vi "Lissajous profiles.vi"() -> ()   [LabVIEW 2021]
panel:
  out "Sine":dynamicdata(graph)
  out "Variance":dynamicdata(graph)
  out "Standard Dev":dynamicdata(graph)
  out "Arithmetic Mean":dynamicdata(graph)
  in  "stop":bool
  in  "Amplitude 2":i32(knob) scale=0.0..10.0
  in  "Amplitude":i32(knob) scale=0.0..10.0
  in  "Phase 2":i32(knob) scale=0.0..50.0
  in  "Phase":i32(knob) scale=0.0..50.0
  in  "Frequency 2":i32(knob) scale=0.0..50.0
  in  "Frequency":i32(knob) scale=0.0..50.0
  out "Lissajous Graph":cluster{"Y":dbl[], "Y":dbl[]}[](graph)
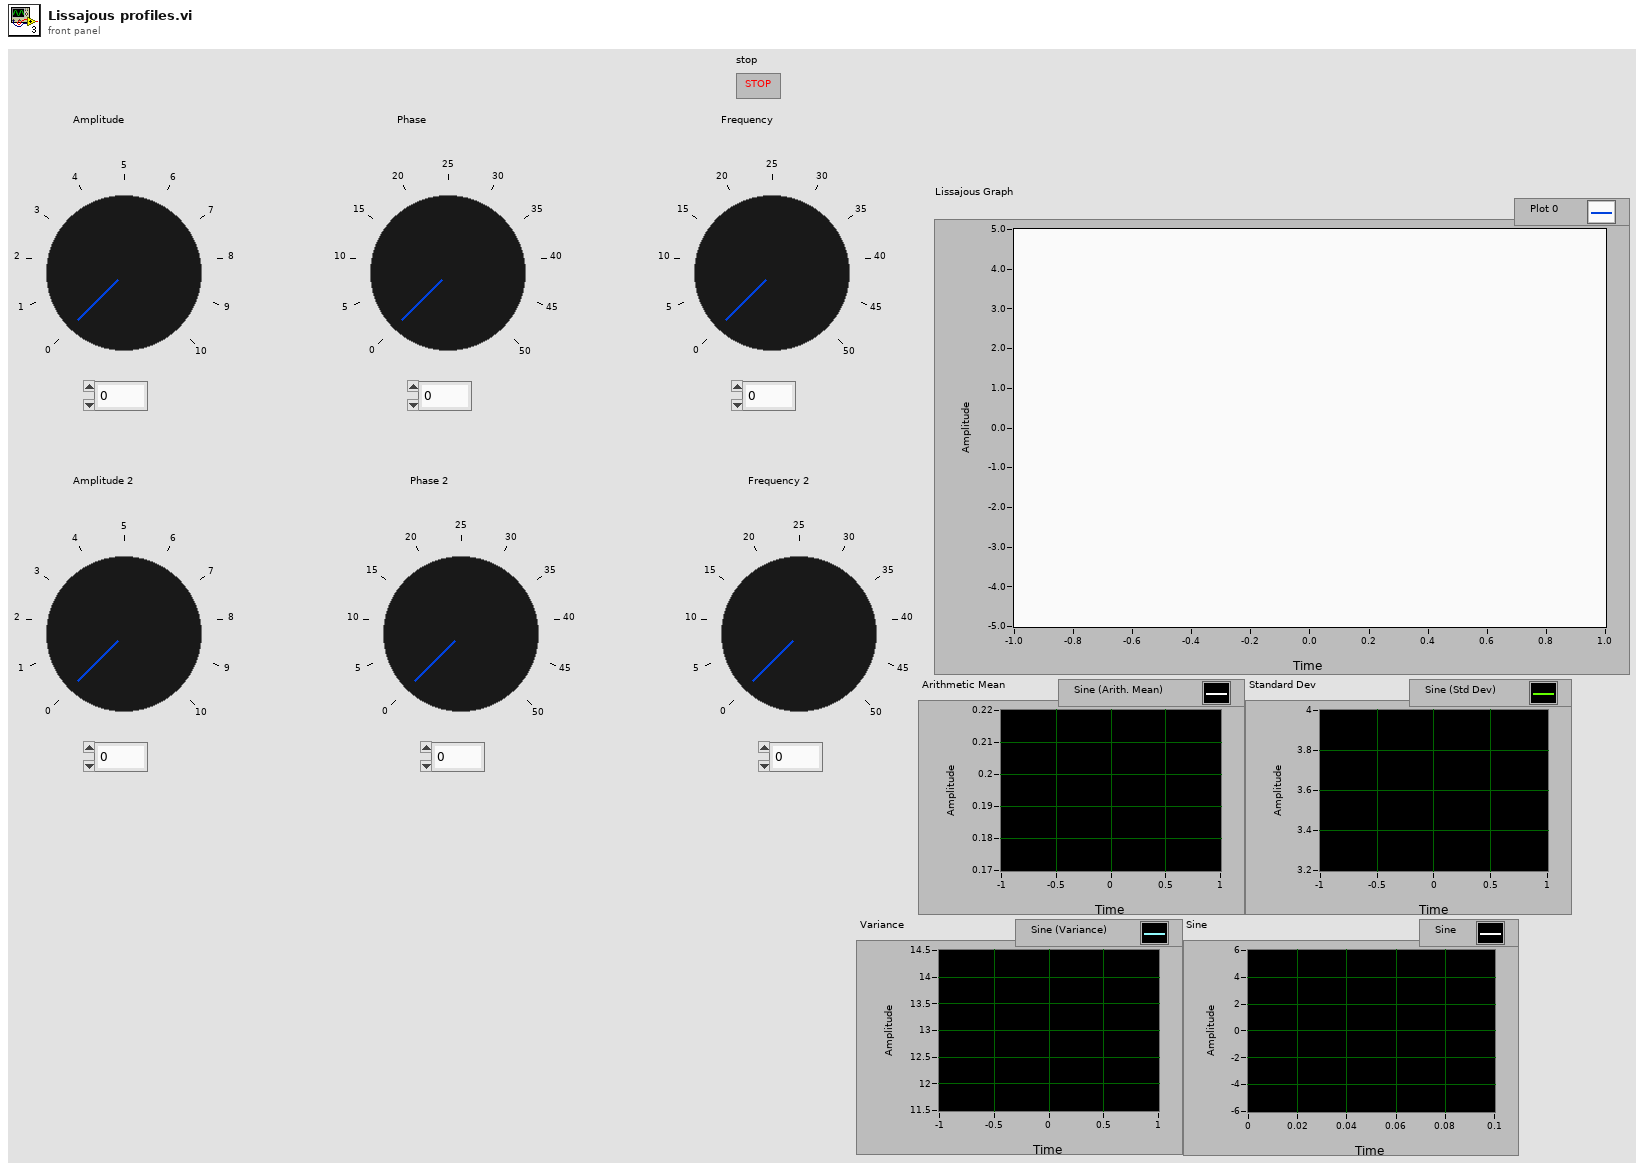
[diagram p1: front panel]
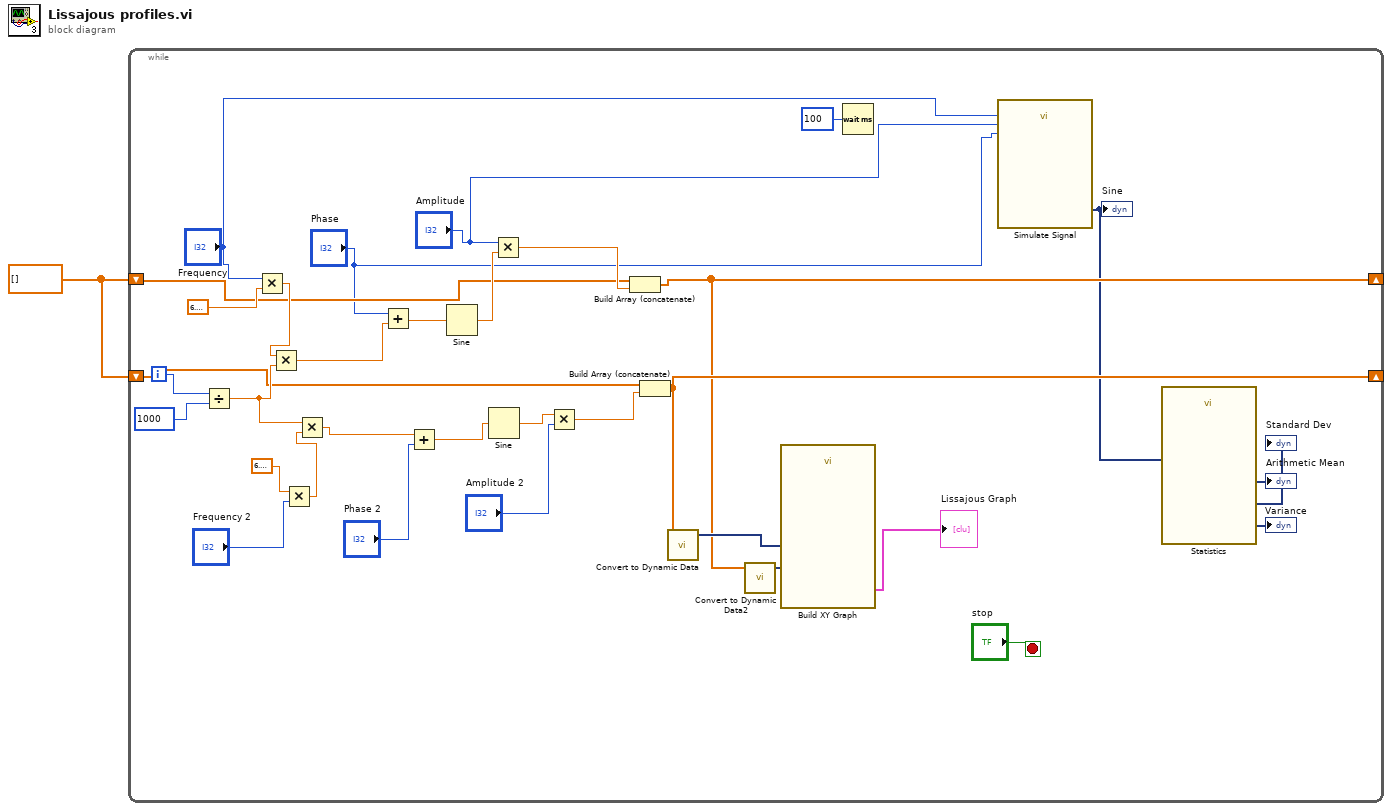
[diagram p0: block diagram]
diagram:
  w1 = dbl[] []
  n1 = while {
    shift-right: [w13] -> _
    shift-left: w1 -> [w18]
    shift-right: [w15] -> _
    shift-left: w1 -> [w16]
    i -> [w34]
    stop <- "stop" stop-if-true
    n2 = Divide(x=w34, y=1000) -> (x/y=w26:dbl)
    n3 = Multiply(x="Frequency", y=6.283185307179586) -> (x*y=w32:dbl)
    n4 = Multiply(x=w32, y=w26) -> (x*y=w31:dbl)
    n5 = Multiply(x=6.283185307179586, y="Frequency 2") -> (x*y=w25:dbl)
    n6 = Multiply(x=w26, y=w25) -> (x*y=w24:dbl)
    n7 = Add(x="Phase", y=w31) -> (x+y=w30:dbl)
    n8 = Add(x=w24, y="Phase 2") -> (x+y=w22:dbl)
    n9 = Sine(x=w30) -> (sin(x)=w29:dbl)
    n10 = Sine(x=w22) -> (sin(x)=w21:dbl)
    n11 = Multiply(x="Amplitude", y=w29) -> (x*y=w19:dbl)
    n12 = Multiply(x=w21, y="Amplitude 2") -> (x*y=w17:dbl)
    n13 = Build Array (concatenate)(w18, w19) -> (w13:dbl[])
    n14 = Build Array (concatenate)(w16, w17) -> (w15:dbl[])
    n15 = call "Convert to Dynamic Data"("Array"=w15) -> ("Dynamic Data Type"=w14:dynamicdata)  [unwired: 3 in]
    n16 = call "Convert to Dynamic Data2"("Array"=w13) -> ("Dynamic Data Type"=w12:dynamicdata)  [unwired: 3 in]
    n17 = call "Build XY Graph"("Y Input"=w12, "X Input"=w14) -> ("XY Graph"=→"Lissajous Graph":cluster{"X":dbl[], "Y":dbl[]}[])  [unwired: 8 in, 1 out]
    n18 = Wait (ms)(milliseconds to wait=u32 100) -> ()  [unwired: 1 out]
    n19 = call "Simulate Signal"("Frequency"="Frequency", "Amplitude"="Amplitude", "Phase"="Phase") -> ("Sine"=w5:dynamicdata)  [unwired: 11 in, 1 out]
    "Sine" <- w5
    n20 = call "Statistics"("Signals"=w5) -> ("Variance"=→"Variance":dynamicdata, "Standard Dev"=→"Standard Dev":dynamicdata, "Arithmetic Mean"=→"Arithmetic Mean":dynamicdata)  [unwired: 23 in, 1 out]
  }
